vi "Freq Band - Divide by Max Bandwidth.vi"(7 "Max Segment Size (100MHz)":dbl=100.0, 11 "Freq Range":cluster{"Fstart":dbl, "Fstop":dbl, "Fstep":dbl}) -> (3 "Sub-Bands":T1(array[cluster]))   [LabVIEW 2011]
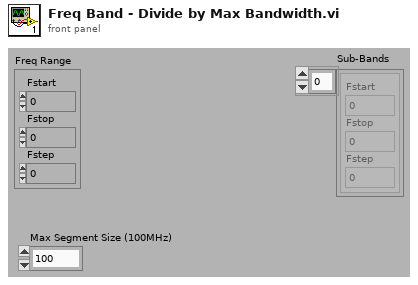
[diagram p1: front panel]
types:
  T1 = cluster{"Fstart":dbl, "Fstop":dbl, "Fstep":dbl}[]
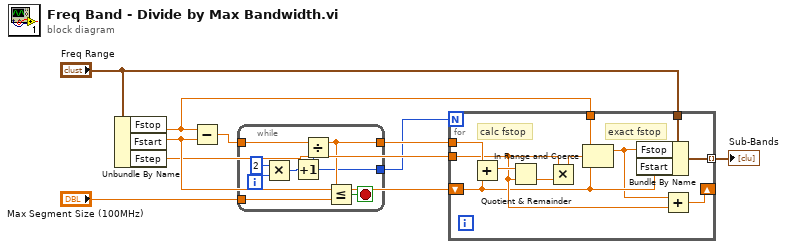
[diagram p0: block diagram]
diagram:
  n1 = Unbundle By Name("Freq Range") -> ("Fstop"=w1:dbl, "Fstart"=w6:dbl, "Fstep"=w5:dbl)
  n2 = Subtract(x=w1, y=w6) -> (x-y=w8:dbl)
  n3 = while {
    tunnel: "Max Segment Size (100MHz)" -> [w17]
    tunnel: w8 -> [w16]
    tunnel: [w11] -> w7
    tunnel: [w10] -> w2
    i -> [w14]
    stop <- w15 stop-if-true
    n4 = Multiply(x=2, y=w14) -> (x*y=w12:i32)
    n5 = Increment(x=w12) -> (x+1=w10:i32)
    n6 = Divide(x=w16, y=w10) -> (x/y=w11:dbl)
    n7 = Less Or Equal?(x=w11, y=w17) -> (x <= y?=w15:bool)
  }
  n8 = for {
    N: w2 -> [_]
    tunnel: w7 -> [w28]
    tunnel: w5 -> [w22]
    shift-right: [w24] -> _
    shift-left: w6 -> [w20]
    tunnel: "Freq Range" -> [w27]
    tunnel: [w23] -> w3 mode=indexing
    tunnel: w1 -> [w21]
    # "exact fstop"
    # "calc fstop"
    n9 = Add(x=w28, y=w20) -> (x+y=w26:dbl)
    n10 = Quotient & Remainder(x=w26, y=w22) -> (floor(x/y)=w25:dbl)  [unwired: 1 out]
    n11 = Multiply(x=w22, y=w25) -> (x*y=w18:dbl)
    n12 = In Range and Coerce(upper limit=w21, x=w18, lower limit=w20) -> (coerced(x)=w19:dbl)  [unwired: 1 out]
    n13 = Bundle By Name(cluster=w27, "Fstop"=w19, "Fstart"=w20) -> (w23:cluster{"Fstart":dbl, "Fstop":dbl, "Fstep":dbl})
    n14 = Add(x=w19, y=w22) -> (x+y=w24:dbl)
  }
  "Sub-Bands" <- w3
